vi "Test.vi"   [LabVIEW 2015]
doc: "This VI is called when test mode begins, and will automatically be terminated when it ends. You can add manual or automatic tests and invoke them from the dashboard."
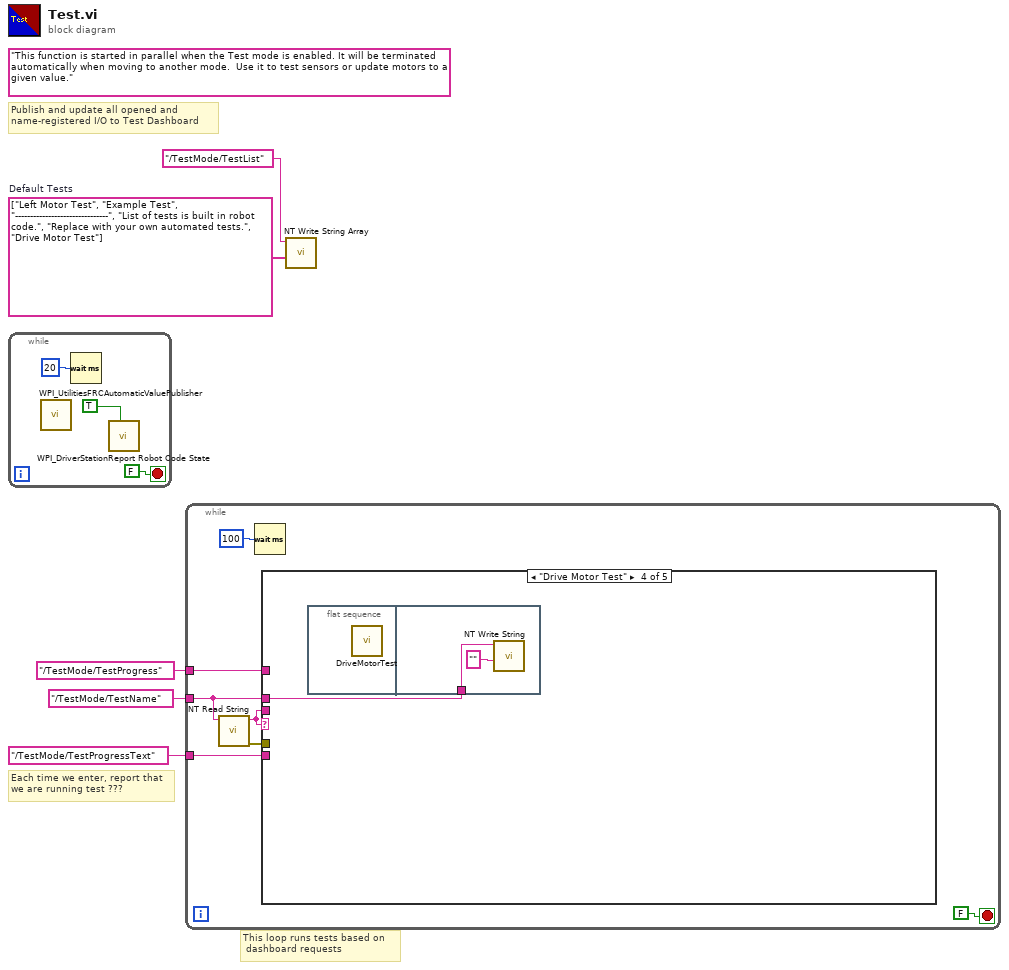
[diagram p0: block diagram]
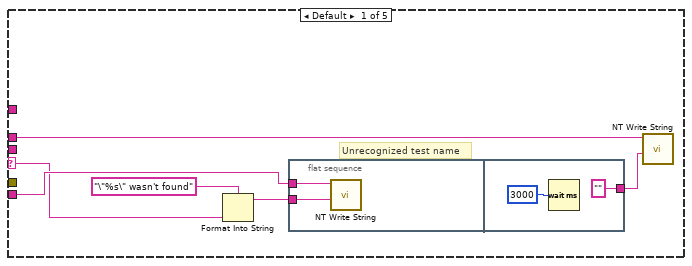
[diagram p2: hidden frame]
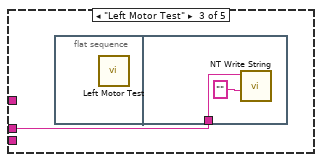
[diagram p4: hidden frame]
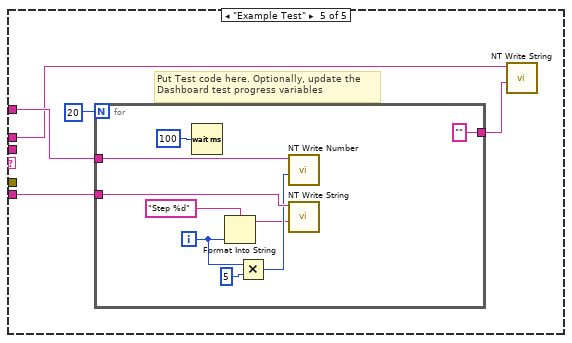
[diagram p5: hidden frame]
diagram:
  w2 = string[] ["Left Motor Test", "Example Test", "-------------------------------", "List of tests is built in robot code.", "Replace with your own automated tests.", "Drive Motor Test"]  # Default Tests
  (unwired) "This function is started in parallel when the Test mode is enabled. It will be terminated automatically when moving to another mode.  Use it to test sensors or update motors to a given value."
  # "This loop runs tests based on \n dashboard requests"
  # "Publish and update all opened and\nname-registered I/O to Test Dashboard"
  # "Each time we enter, report that\nwe are running test ???"
  n1 = while {
    stop <- FALSE stop-if-true
    n2 = call <vilib>:"WPI_UtilitiesFRCAutomaticValuePublisher.vi"() -> ()  [unwired: 12 in]
    n3 = Wait (ms)(milliseconds to wait=u32 20) -> ()  [unwired: 1 out]
    n4 = call <vilib>:"WPI_DriverStationReport Robot Code State.vi"("Test"=TRUE ("Autonomous")) -> ()  [unwired: 10 in, 1 out]
  }
  n5 = while {
    tunnel: "/TestMode/TestName" ("Name") -> [w10]
    tunnel: "/TestMode/TestProgressText" ("Name") -> [w13]
    tunnel: "/TestMode/TestProgress" ("Name") -> [w12]
    stop <- FALSE stop-if-true
    n6 = call <vilib>:"NT Read String.vi"("Name"=w10) -> ("error out"=w9:errorcluster, "String"=w11:string)  [unwired: 9 in]
    n7 = Wait (ms)(milliseconds to wait=u32 100) -> ()  [unwired: 1 out]
    n8 = case shown="\"Drive Motor Test\"" w11 {
      selector: w11 -> [w20 _ _ _ _]
      tunnel: w10 -> [w17 _ w26 w29 w32]
      tunnel: w13 -> [w21 _ _ _ w35]
      tunnel: w12 -> [_ _ _ _ w36]
      tunnel: w11 -> [_ _ _ _ _]
      tunnel: w9 -> [_ _ _ _ _]
      frame Default {
        # "Unrecognized test name"
        n9 = Format Into String(format string="\"%s\" wasn't found" ("Name"), w20) -> (resulting string=w19:string)  [unwired: 2 in, 1 out]
        n10 = flat-sequence {
          tunnel: w21 -> [w22]
          tunnel: w19 -> [w23]
          tunnel: ["" ("Name")] -> w16
          frame #0 {
            n11 = call <vilib>:"NT Write String.vi"("String"=w23, "Name"=w22) -> ()  [unwired: 9 in, 1 out]
          }
          frame #1 {
            n12 = Wait (ms)(milliseconds to wait=u32 3000) -> ()  [unwired: 1 out]
          }
        }
        n13 = call <vilib>:"NT Write String.vi"("String"=w16, "Name"=w17) -> ()  [unwired: 9 in, 1 out]
      }
      frame "" {
        # "No test to run"
      }
      frame "Left Motor Test" {
        n14 = flat-sequence {
          tunnel: w26 -> [w28]
          frame #0 {
            n15 = call "Left Motor Test.vi"() -> ()  [unwired: 12 in]
          }
          frame #1 {
            n16 = call <vilib>:"NT Write String.vi"("String"="", "Name"=w28) -> ()  [unwired: 9 in, 1 out]
          }
        }
      }
      frame "Drive Motor Test" {
        n17 = flat-sequence {
          tunnel: w29 -> [w31]
          frame #0 {
            n18 = call "DriveMotorTest.vi"() -> ()  [unwired: 12 in]
          }
          frame #1 {
            n19 = call <vilib>:"NT Write String.vi"("String"="", "Name"=w31) -> ()  [unwired: 9 in, 1 out]
          }
        }
      }
      frame "Example Test" {
        # "Put Test code here. Optionally, update the\nDashboard test progress variables"
        n20 = for {
          N: 20 -> [_]
          tunnel: w36 -> [w45]
          tunnel: w35 -> [w43]
          tunnel: ["" ("String")] -> w33
          i -> [w40]
          n21 = Wait (ms)(milliseconds to wait=u32 100) -> ()  [unwired: 1 out]
          n22 = Format Into String(format string="Step %d", w40) -> (resulting string=w38:string)  [unwired: 2 in, 1 out]
          n23 = Multiply(x=w40, y=u32 5 ("milliseconds to wait")) -> (x*y=w41:u32)
          n24 = call <vilib>:"NT Write Number.vi"("Numeric"=w41, "Name"=w45) -> ()  [unwired: 9 in, 1 out]
          n25 = call <vilib>:"NT Write String.vi"("String"=w38, "Name"=w43) -> ()  [unwired: 9 in, 1 out]
        }
        n26 = call <vilib>:"NT Write String.vi"("String"=w33, "Name"=w32) -> ()  [unwired: 9 in, 1 out]
      }
    }
  }
  n27 = call <vilib>:"NT Write String Array.vi"("String Array"=w2, "Name"="/TestMode/TestList") -> ()  [unwired: 9 in, 1 out]
